vi "Read Shared Variables - SuNLaMP RTD 4.vi"(9 "channel errors in (no errors)":errorcluster[](array[cluster])) -> (1 "channel errors out":errorcluster[](array[cluster]), 2 "data":dbl[](array[numeric]), 3 "UUIDs":string[](array[string])=["Flow Rate [g/s]", "Density [g/cm^3]", "Return Filter dP [psid]", "Outlet Filter and Flowmeter dp [psid]", "Cooler dP [psid]", "Cooler CO2 In [F]", "Cooler CO2 Out [F]", "Pump Frequency [%]", "Recirc Valve Open [%]"])   [LabVIEW 2020]
uses:
  <vilib>/Utility/error.llb/Error Cluster From Error Code.vi
  <vilib>/ErrorRing/Error Ring.xnode
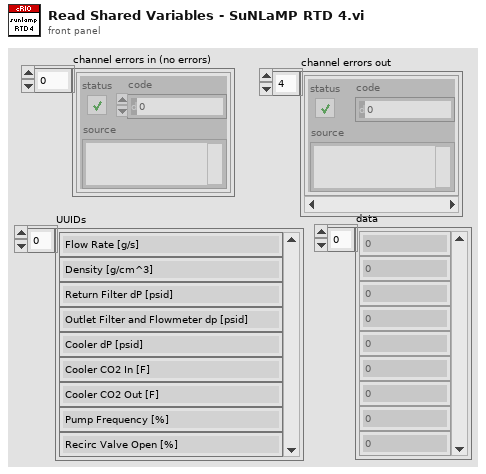
[diagram p1: front panel]
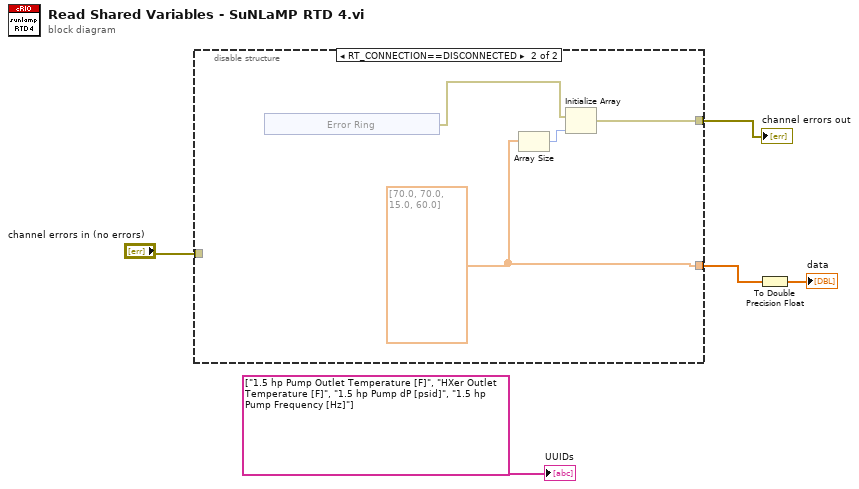
[diagram p0: block diagram]
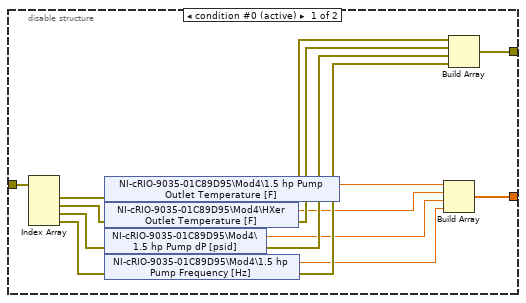
[diagram p2: hidden frame]
diagram:
  n1 = disable-structure shown="RT_CONNECTION==DISCONNECTED" {
    disable-tunnel: [w12 w22] -> w4
    disable-tunnel: "channel errors in (no errors)" -> [w11 _]
    disable-tunnel: [w6 w21] -> w1
    frame condition #0 (active) {
      n2 = Index Array(array=w11) -> (element #1=w10:errorcluster, element #2=w9:errorcluster, element #3=w8:errorcluster, element #4=w7:errorcluster)  [unwired: 4 in]
      n3 = shared-variable "NI-cRIO-9035-01C89D95\\Mod4\\1.5 hp Pump Outlet Temperature [F]"(error in=w10) -> (w13:dbl, error out=w17:errorcluster)
      n4 = shared-variable "NI-cRIO-9035-01C89D95\\Mod4\\HXer Outlet Temperature [F]"(error in=w9) -> (w14:dbl, error out=w18:errorcluster)
      n5 = shared-variable "NI-cRIO-9035-01C89D95\\Mod4\\1.5 hp Pump dP [psid]"(error in=w8) -> (w15:dbl, error out=w19:errorcluster)
      n6 = shared-variable "NI-cRIO-9035-01C89D95\\Mod4\\1.5 hp Pump Frequency [Hz]"(error in=w7) -> (w16:dbl, error out=w20:errorcluster)
      n7 = Build Array(w13, w14, w15, w16) -> (w6:dbl[])
      n8 = Build Array(w17, w18, w19, w20) -> (w12:errorcluster[])
    }
    frame condition #1 {
      w21 = dbl[] [70.0, 70.0, 15.0, 60.0] ("data")
      n9 = xnode "Error Ring"() -> ("error out"=w23:errorcluster)
      n10 = Array Size(array=w21) -> (size(s)=w24:i32)
      n11 = Initialize Array(w23, w24) -> (w22:errorcluster[])
    }
  }
  "channel errors out" <- w4
  n12 = To Double Precision Float(number=w1) -> (double precision float=→"data":dbl[])
  "UUIDs" <- string[] ["1.5 hp Pump Outlet Temperature [F]", "HXer Outlet Temperature [F]", "1.5 hp Pump dP [psid]", "1.5 hp Pump Frequency [Hz]"]
